vi "Action - DAQ AI Reader.vi"(7 "PackageID":i32, 8 "error in":errorcluster, 10 "DAQ AI Configuration":T1={"AI Channels"="Dev1/ao0", "Min (V)"=-5.0, "Max (V)"=5.0, "Terminal Config"=-1, "Sample Rate (Hz)"=1000.0, "#Samples"=100} {"Terminal Config" items=["Default"=-1, "RSE"=10083, "NRSE"=10078, "Differential"=10106, "Pseudodifferential"=12529]; "Min (V)" format="%#_13g"; "Max (V)" format="%#_13g"; "Sample Rate (Hz)" format="%#_13g"}, 11 "DAQ AI Task":refnum<k21>) -> (0 "error out":errorcluster)   [LabVIEW 2021, in "XNET-CAN-Signal-Logger.lvlib"]
uses:
  XNET-CAN-Signal-Logger.lvlib
  Typedef/Def-DAQ AI Configuration.ctl
  Typedef/Def-Data Queue Type.ctl
  Typedef/Def-GSTOP.ctl
  <vilib>/DAQmx/read.llb/DAQmx Read (Analog 1D Wfm NChan NSamp).vi
  Global Variables.vi
  <userlib>/_NEVSTOP/GlobalStop/_gStop.vi
  <vilib>/DAQmx/miscellaneous.llb/DAQmx Fill In Error Info.vi
  <userlib>/_NEVSTOP/GlobalStop/GSTOP.lvlib
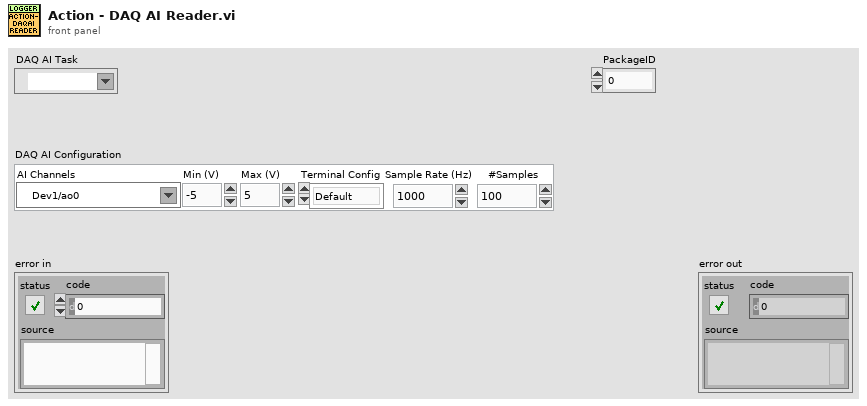
[diagram p1: front panel]
types:
  T1 = typedef "XNET-CAN-Signal-Logger.lvlib/Def-DAQ AI Configuration.ctl" = cluster{"AI Channels":tag, "Min (V)":dbl, "Max (V)":dbl, "Terminal Config":i32, "Sample Rate (Hz)":dbl, "#Samples":i32}
  T2 = typedef "XNET-CAN-Signal-Logger.lvlib/Def-Data Queue Type.ctl" = cluster{"PackageID":i32, "Data":waveform(dbl)[]}
  T3 = typedef "XNET-CAN-Signal-Logger.lvlib/Def-GSTOP.ctl" = enum16{"Writer", "Readers"}
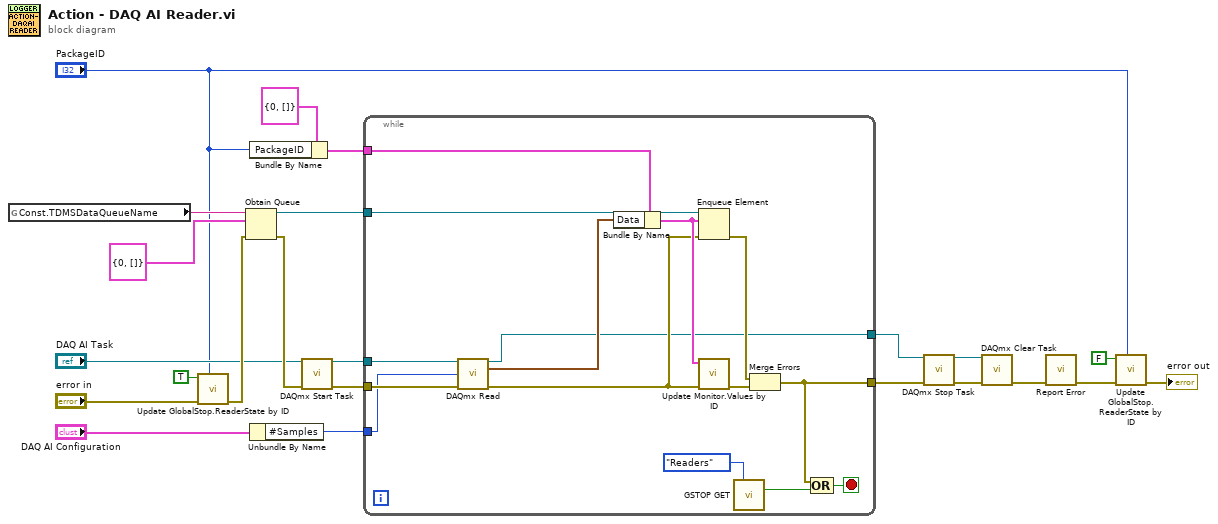
[diagram p0: block diagram]
diagram:
  n1 = global read "Global Variables.vi" "Const.TDMSDataQueueName"() -> (w21:string)
  n2 = call "Update GlobalStop.ReaderState by ID.vi"("PackageID"="PackageID", "error in"="error in", "RunState"=TRUE) -> ("error out"=w5:errorcluster)  [unwired: 8 in]
  n3 = Obtain Queue(name (unnamed)=w21, element data type=T2 {"PackageID"=0, "Data"=[]} ("Data Queue Type"), error in (no error)=w5) -> (queue out=w19:refnum<queue>, error out=w4:errorcluster)  [unwired: 2 in, 1 out]
  n4 = Bundle By Name(cluster=T2 {"PackageID"=0, "Data"=[]} ("element"), "PackageID"="PackageID") -> (w22:T2)
  n5 = Unbundle By Name("DAQ AI Configuration") -> ("#Samples"=w9:i32)
  n6 = call <vilib>:"DAQmx Start Task.vi"("task/channels in"="DAQ AI Task", "error in"=w4) -> ("task out"=w17:refnum<k21>, "error out"=w16:errorcluster)  [unwired: 12 in]
  n7 = while {
    tunnel: w19 -> [w37]
    tunnel: w17 -> [w38]
    tunnel: w16 -> [w34]
    tunnel: w22 -> [w36]
    tunnel: [w28] -> w11
    tunnel: [w27] -> w14
    tunnel: w9 -> [w26]
    stop <- w35 stop-if-true
    n8 = call-poly <vilib>:"DAQmx Read.vi"("task/channels in"=w38, "number of samples per channel"=w26, "error in"=w34) -> ("task out"=w27:refnum<k21>, "data"=w33:waveform(dbl)[], "error out"=w31:errorcluster)  [unwired: 10 in]
    n9 = Bundle By Name(cluster=w36, "Data"=w33) -> (w32:T2)
    n10 = Enqueue Element(queue=w37, element=w32, error in (no error)=w31) -> (error out=w29:errorcluster)  [unwired: 1 in, 2 out]
    n11 = call "Update Monitor.Values by ID.vi"("error in"=w31, "Data"=w32) -> ("error out"=w30:errorcluster)  [unwired: 9 in]
    n12 = call <userlib>:"GSTOP GET.vi"("index(-1 for All)"=Def-GSTOP."Readers" ("GSTOP")) -> ("stop"=w25:bool)  [unwired: 13 in, 1 out]
    n13 = Merge Errors(w29, w30) -> (w28:errorcluster)
    n14 = Compound Arithmetic op=OR(w28, w25) -> (w35:bool)
  }
  n15 = call <vilib>:"DAQmx Stop Task.vi"("task/channels in"=w14, "error in"=w11) -> ("task out"=w15:refnum<k21>, "error out"=w12:errorcluster)  [unwired: 12 in]
  n16 = call <vilib>:"DAQmx Clear Task.vi"("task in"=w15, "error in"=w12) -> ("error out"=w13:errorcluster)  [unwired: 13 in]
  n17 = call "Report Error.vi"("error in (no error)"=w13) -> ("error out"=w18:errorcluster)  [unwired: 10 in]
  n18 = call "Update GlobalStop.ReaderState by ID.vi"("PackageID"="PackageID", "error in"=w18, "RunState"=FALSE) -> ("error out"=→"error out":errorcluster)  [unwired: 8 in]
